vi "003 Crea array aleatori i inverteix.vi"() -> ()   [LabVIEW 2019]
uses:
  <vilib>/numeric/Random Number (Range) DBL.vi
panel:
  out "Array invertit":dbl[](array[numeric])
  out "Array 10 pos\nnombre aleatoris":dbl[](array[numeric])
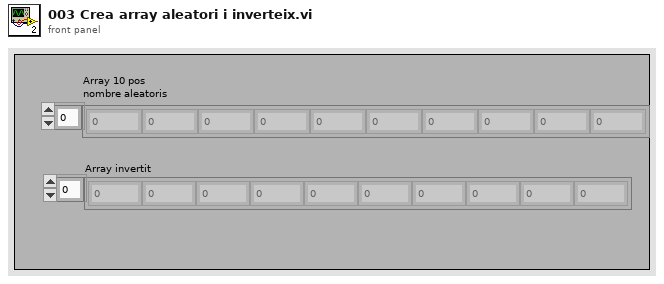
[diagram p1: front panel]
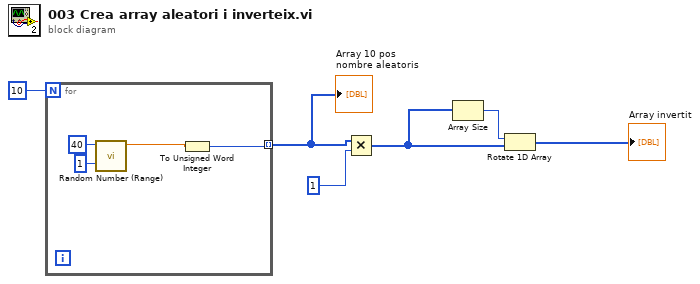
[diagram p0: block diagram]
diagram:
  n1 = for {
    N: 10 -> [_]
    tunnel: [w7] -> w5 mode=indexing
    n2 = call-poly <vilib>:"Random Number (Range).vi"("lower bound (0)"=u64 1, "upper bound (100)"=u64 40) -> ("number"=w8:dbl)  [unwired: 9 in]
    n3 = To Unsigned Word Integer(number=w8) -> (unsigned 16bit integer=w7:u16)
  }
  "Array 10 pos\nnombre aleatoris" <- w5
  n4 = Multiply(x=w5, y=1) -> (x*y=w2:i32[])
  n5 = Array Size(array=w2) -> (size(s)=w1:i32)
  n6 = Rotate 1D Array(1:w2, 2:w1) -> (0:→"Array invertit":i32[])
